vi "项名.vi"(8 "error in (no error)":errorcluster caption="错误输入（无错误）", 11 "Copy 输入":refnum<class "Copy.lvclass">) -> (0 "error out":errorcluster caption="错误输出", 3 "Copy 输出":refnum<class "Copy.lvclass">)   [LabVIEW 2016, in "Copy.lvclass"]
uses:
  Copy.lvclass
  Parent Class/Menu.lvclass
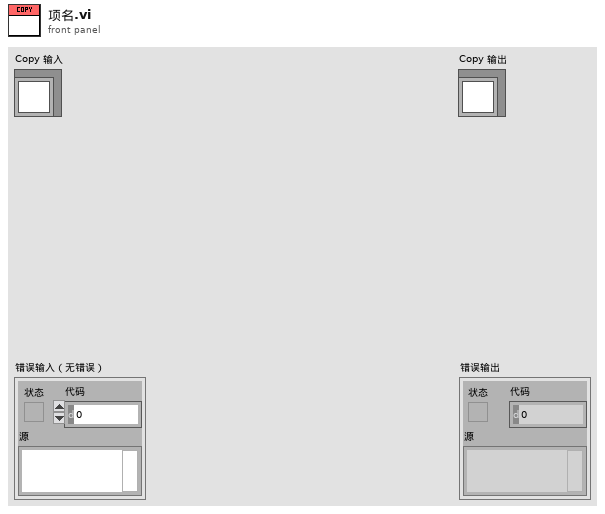
[diagram p1: front panel]
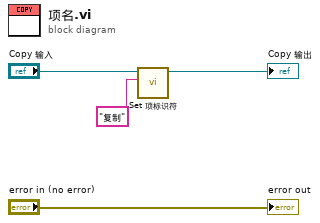
[diagram p0: block diagram]
diagram:
  n1 = call "Set 项标识符.vi"("项标识符"="复制", "LNK in"="Copy 输入") -> ("LNK out"=→"Copy 输出":refnum<class "Copy.lvclass">)  [unwired: 9 in]
  "error out" <- "error in (no error)"
